vi "GetAvailableInteractions.vi"(8 "error in (no error)":errorcluster, 11 "Topas In":refnum<k24>) -> (0 "error out":errorcluster, 2 "Available interactions":cluster{"Type":string, "From":dbl, "To":dbl}[](array[cluster]), 3 "Topas out":refnum<k24>)   [LabVIEW 2017]
uses:
  D:/upwork/Laser Measurement Tool/Topas4PublicAPI/NET_SDK/Topas4Lib.dll
  Topas4PublicAPI/NET_SDK/Topas4Lib.dll
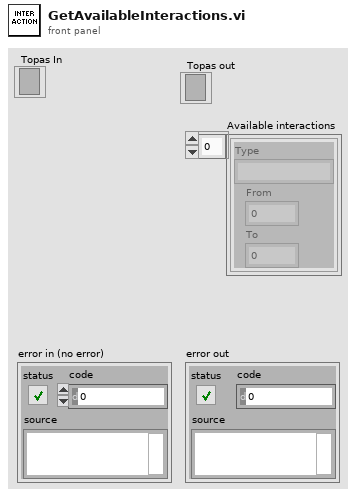
[diagram p1: front panel]
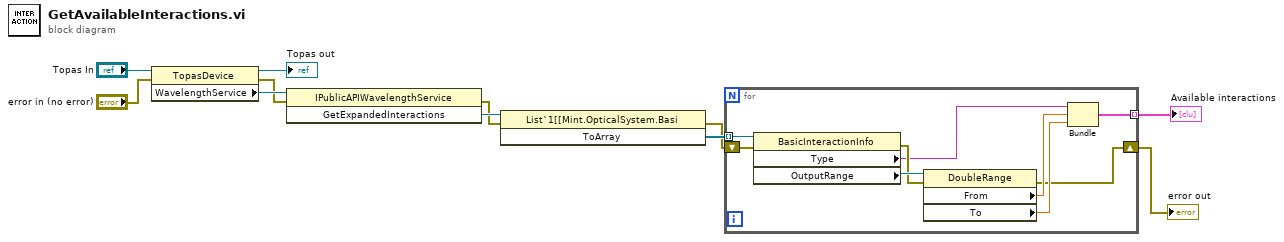
[diagram p0: block diagram]
diagram:
  n1 = property class="TopasDevice"(reference="Topas In", error in="error in (no error)") -> (reference out=→"Topas out":refnum<k24>, error out=w7:errorcluster, "WavelengthService"=w9:refnum<k24>)
  n2 = invoke class="IPublicAPIWavelengthService" method="GetExpandedInteractions"(reference=w9, error in=w7) -> (error out=w5:errorcluster, "GetExpandedInteractions"=w10:refnum<k24>)  [unwired: 1 in, 1 out]
  n3 = invoke class="List`1[[Mint.OpticalSystem.Basi" method="ToArray"(reference=w10, error in=w5) -> (error out=w4:errorcluster, "ToArray"=w11:refnum<k24>[])  [unwired: 1 in, 1 out]
  n4 = for {
    tunnel: w11 -> [w20] mode=indexing
    shift-right: [w13] -> w3
    shift-left: w4 -> [w18]
    tunnel: [w12] -> w1 mode=indexing
    n5 = property class="BasicInteractionInfo"(reference=w20, error in=w18) -> (error out=w17:errorcluster, "Type"=w16:string, "OutputRange"=w19:refnum<k24>)  [unwired: 1 out]
    n6 = property class="DoubleRange"(reference=w19, error in=w17) -> (error out=w13:errorcluster, "From"=w15:dbl, "To"=w14:dbl)  [unwired: 1 out]
    n7 = Bundle("Type"=w16, "From"=w15, "To"=w14) -> (w12:cluster{"Type":string, "From":dbl, "To":dbl})  [unwired: 1 in]
  }
  "error out" <- w3
  "Available interactions" <- w1
